vi "Rangemap_Vi_BM_envelope_Huan_4.vi"(0 "inputIR":dbl[](array[numeric])=array[10000 elements], 1 "winkel":dbl=107.5, 2 "correctionValue(samples)":dbl, 3 "distance from origin(cm) X":dbl format="%#_13g", 4 "Gap(samples)":dbl=41.0, 5 "RangeMap":dbl[][](array[numeric])=array200x300[60000 elements], 6 "MaxtPeak miltiplication factor":dbl=25.0, 7 "distance from origin(cm) Y":dbl format="%#_13g", 9 "Datenbank?":bool=TRUE, 10 "Grenz Ampulitude":dbl=80.0, 11 "Pfad-Datenbank":path=path "C:/Users/Administrator/Documents/New LabView Programms/Aktuelle Programme/Experiment!/HuanSubVIs/S35-10_M1.csv", 13 "Wechle Lautsprecher?":i32=11, 18 "Sigma":dbl=2.0) -> (12 "Locations":dbl[](array[numeric]), 14 "OutputRangeMap1":dbl[][](array[numeric]), 17 "distanceMatrix":dbl[][](array[numeric]), 19 "OutputRangeMap2":dbl[][](array[numeric]))   [LabVIEW 2014]
uses:
  <vilib>/Analysis/3filter.llb/Filter Passband Type.ctl
  <vilib>/Analysis/3filter.llb/Butterworth Filter (DBL).vi
  <vilib>/Analysis/NI_AALBase.lvlib
panel:
  out "Element x":i32
  out "Element y":i32
  out "Impulsantwort (gemittelt)":dbl[][](graph)
  in  "RMS miutiplication factor":dbl=3.0
  in  "Noise Level":dbl=4.0
  out "FirstGap":dbl
  out "Array 2":dbl[](array[numeric])
  out "HS":bool
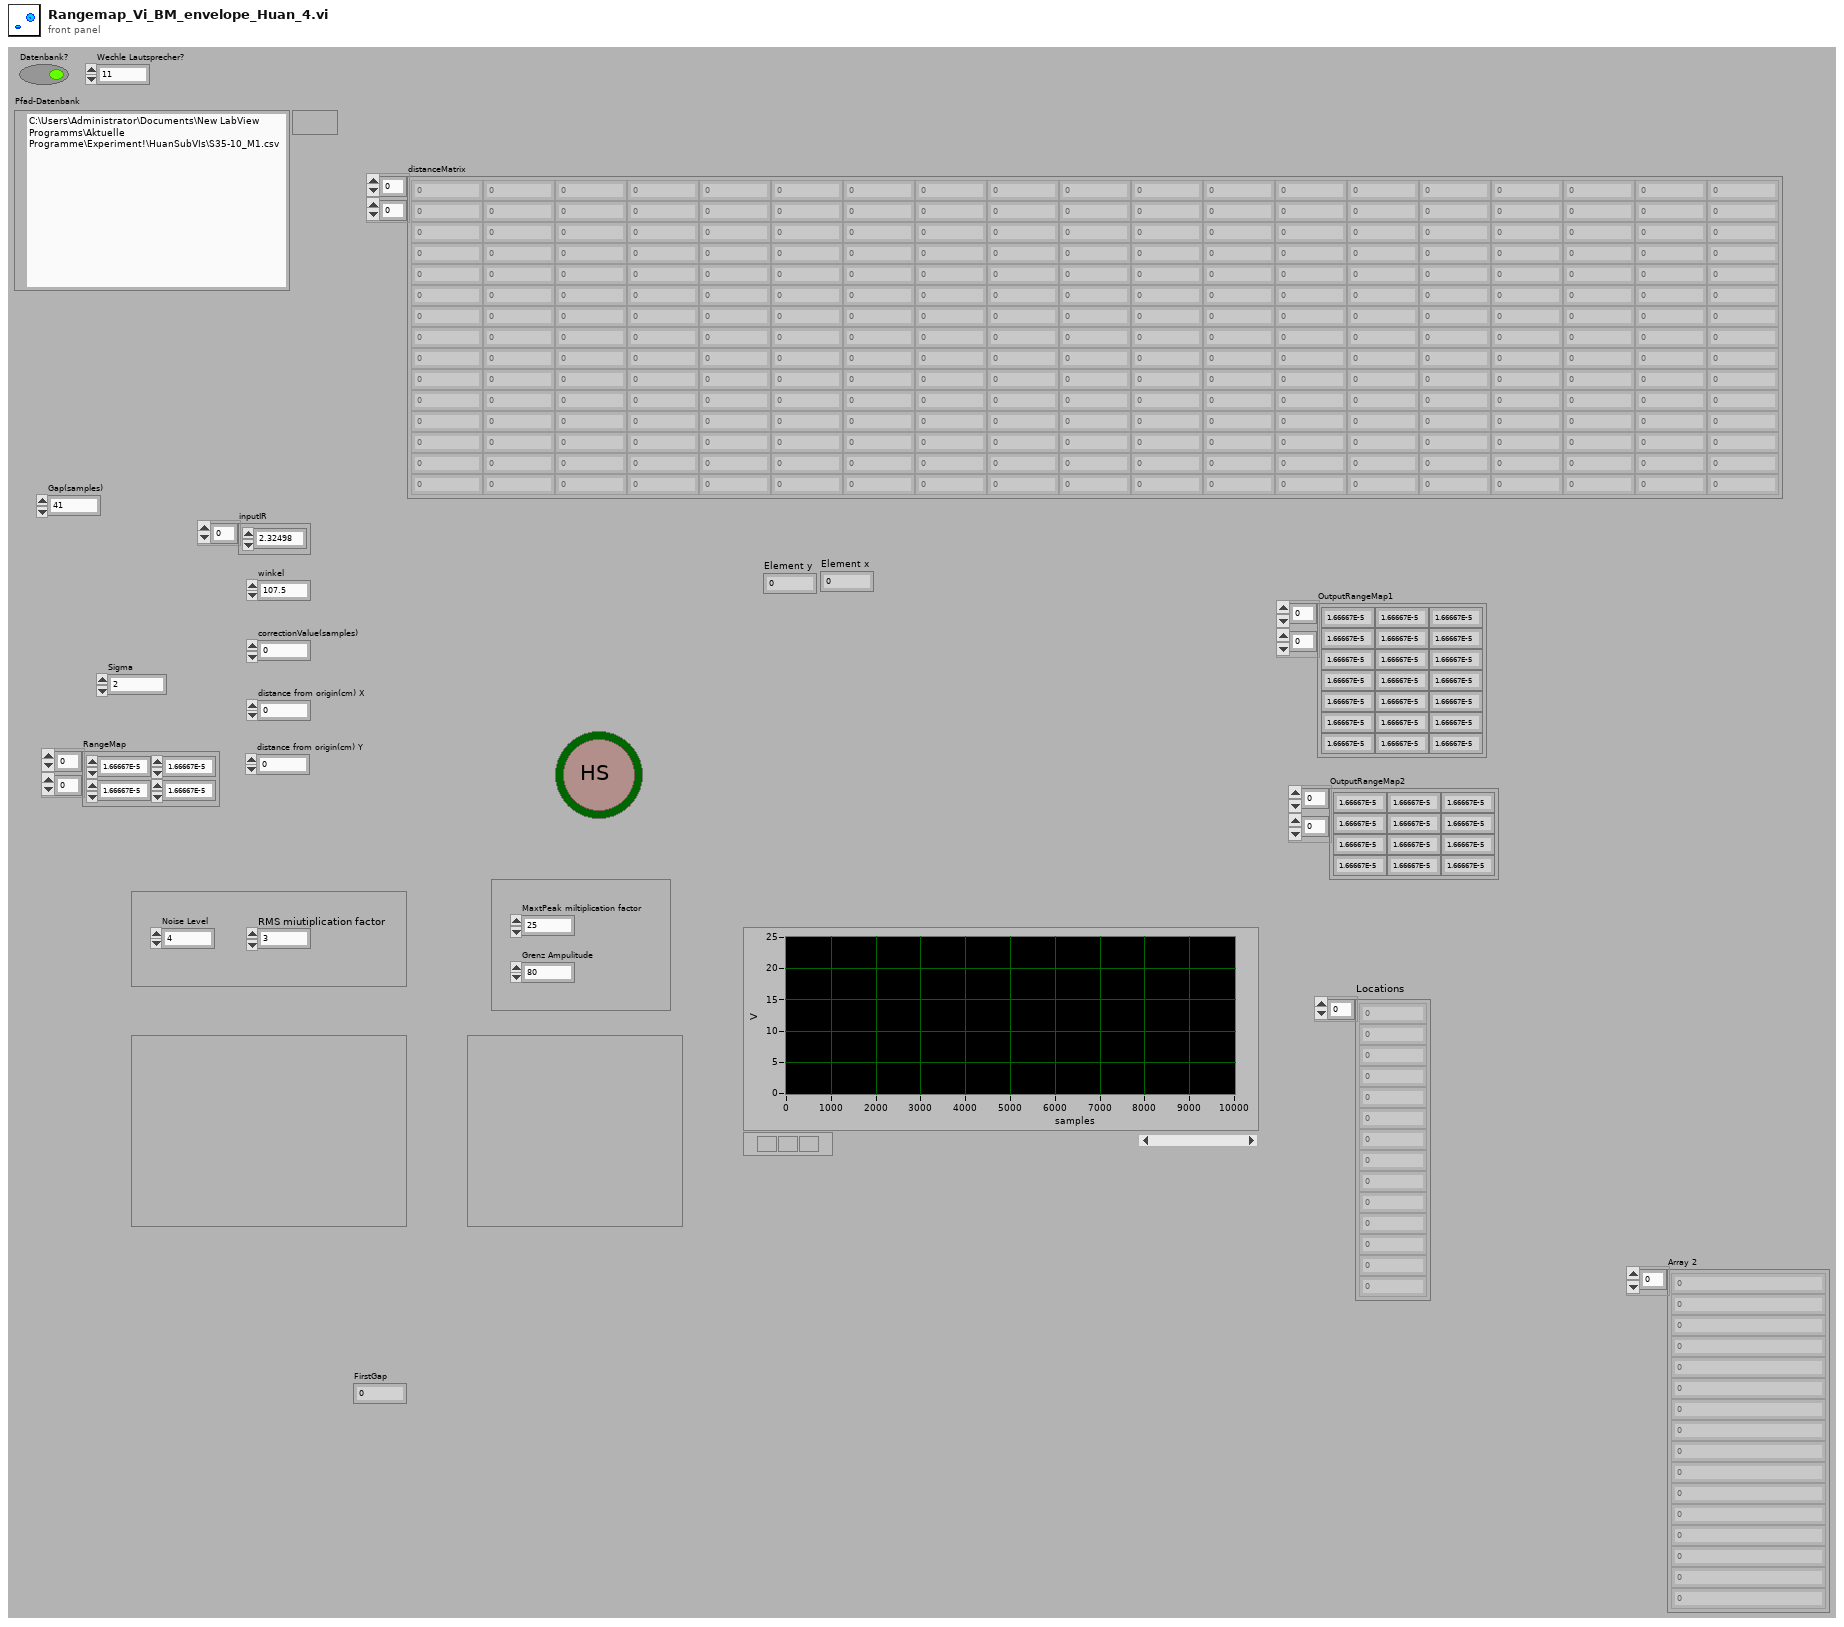
[diagram p1: front panel]
types:
  T1 = typedef "NI_AALBase.lvlib/Filter Passband Type.ctl" = enum32{"Lowpass", "Highpass", "Bandpass", "Bandstop"}
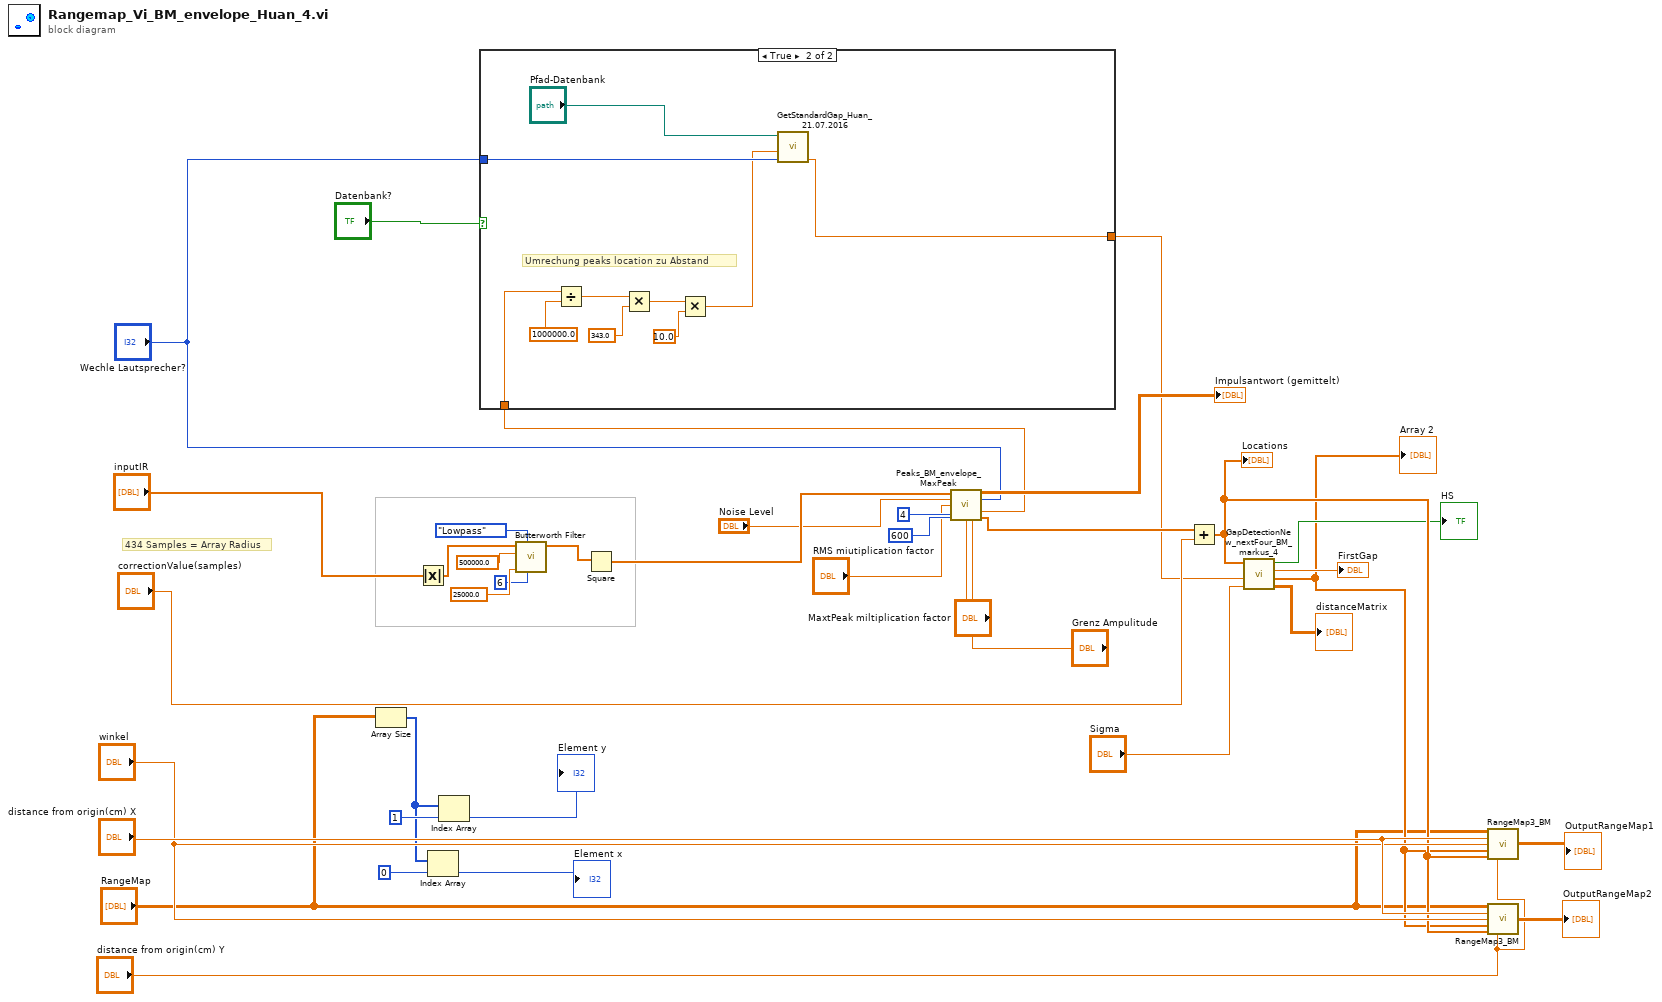
[diagram p0: block diagram]
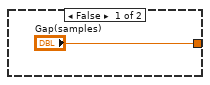
[diagram p2: hidden frame]
diagram:
  # "434 Samples = Array Radius"
  n1 = Array Size(array="RangeMap") -> (size(s)=w2:i32[])
  n2 = Absolute Value(x="inputIR") -> (abs(x)=w29:dbl[])
  n3 = Index Array(array=w2, index=0 ("Index")) -> (element=→"Element x":i32)
  n4 = Index Array(array=w2, index=1 ("Index")) -> (element=→"Element y":i32)
  n5 = call-poly <vilib>:"Butterworth Filter.vi"("order"=6, "filter type"=Filter_Passband_Type."Lowpass", "low cutoff freq: fl"=25000.0 ("high cutoff freq: fh"), "sampling freq: fs"=500000.0, "X"=w29) -> ("Filtered X"=w28:dbl[])  [unwired: 3 in, 1 out]
  n6 = Square(x=w28) -> (x^2=w25:dbl[])
  n7 = call "Peaks_BM_envelope_MaxPeak.vi"("imput sequence"=w25, "Noise Level"="Noise Level", "welche LS ?"="Wechle Lautsprecher?", "RMS miutiplication factor"="RMS miutiplication factor", "width 1"=4 ("width"), "Length of Lsimp"=600, "MaxPeak miltiplication factor"="MaxtPeak miltiplication factor", "Grenz Ampulitude"="Grenz Ampulitude") -> ("IR with theshold"=→"Impulsantwort (gemittelt)":dbl[][], "FirstPeak"=w10:dbl, "Peak Locations"=w23:dbl[])  [unwired: 5 in]
  n8 = case shown="True" "Datenbank?" {
    tunnel: ["Gap(samples)" w40] -> w12
    tunnel: "Wechle Lautsprecher?" -> [_ w48]
    tunnel: w10 -> [_ w47]
    frame False {
    }
    frame True {
      # "Umrechung peaks location zu Abstand"
      n9 = Divide(x=w47, y=1000000.0) -> (x/y=w45:dbl)
      n10 = Multiply(x=w45, y=343.0) -> (x*y=w43:dbl)
      n11 = Multiply(x=w43, y=10.0) -> (x*y=w41:dbl)
      n12 = call "GetStandardGap_Huan_21.07.2016.vi"("Welcher Lautsprecher?"=w48, "Distance in dm"=w41, "Pfad-Datenbank"="Pfad-Datenbank") -> ("Standard Gap"=w40:dbl)  [unwired: 7 in, 1 out]
    }
  }
  n13 = Add(x=w23, y="correctionValue(samples)") -> (x+y=w18:dbl[])
  "Locations" <- w18
  n14 = call "GapDetectionNew_nextFour_BM_markus_4.vi"("Sigma in Prozent"="Sigma", "Gap"=w12, "Locations"=w18) -> ("distanceMatrix"=→"distanceMatrix":dbl[][], "Array"=w15:dbl[], "FirstGap"=→"FirstGap":dbl, "GapPresent"=→"HS":bool)  [unwired: 5 in]
  "Array 2" <- w15
  n15 = call "RangeMap3_BM.vi"("InputArray"="RangeMap", "distance from origin(cm) X"="distance from origin(cm) X", "angle"="winkel", "probablities"=w15, "indices"=w18, "distance from origin(cm) Y"="distance from origin(cm) Y") -> ("OutputArray"=→"OutputRangeMap1":dbl[][])  [unwired: 7 in, 2 out]
  n16 = call "RangeMap3_BM.vi"("InputArray"="RangeMap", "distance from origin(cm) X"="distance from origin(cm) X", "angle"="winkel", "probablities"=w15, "indices"=w18, "distance from origin(cm) Y"="distance from origin(cm) Y") -> ("OutputArray"=→"OutputRangeMap2":dbl[][])  [unwired: 7 in, 2 out]
